vi "InstrumentCalibration - Remove Channel (SubVI).vi"(8 "error in":errorcluster, 11 "Table":string[][](array[string])) -> (0 "error out":errorcluster, 2 "Cancel out":bool, 3 "index":u16)   [LabVIEW 2019]
uses:
  Controls/FGV States.ctl
panel:
  in  "Cancel":bool
  in  "Ok":bool
  in  "Channel to Remove":u16(ring)
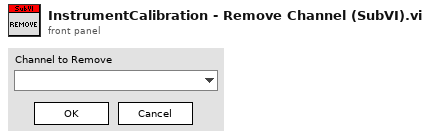
[diagram p1: front panel]
types:
  T1 = typedef "FGV States.ctl" = enum16{"Read", "Write"}
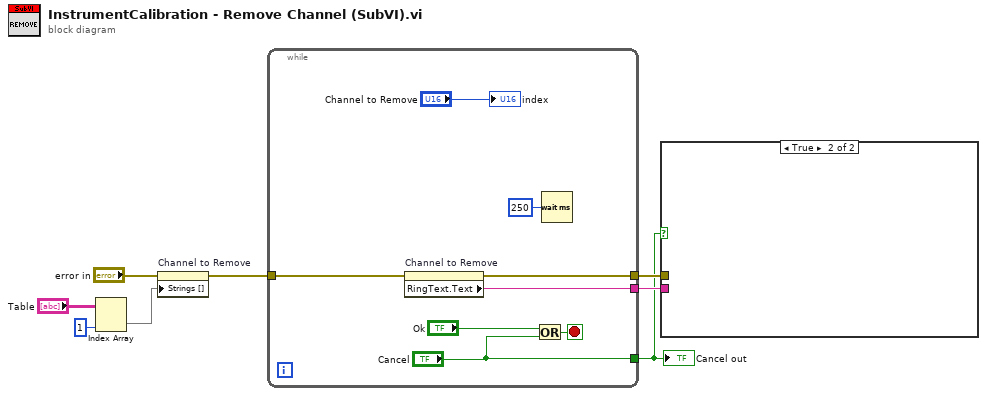
[diagram p0: block diagram]
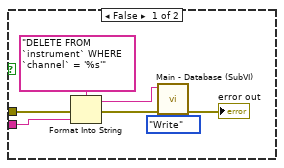
[diagram p2: hidden frame]
diagram:
  n1 = Index Array(array="Table", index (col)=1 ("disabled index (col)")) -> (element=w4:string[])  [unwired: 1 in]
  n2 = property on="Channel to Remove" class="Ring (strict)"(error in="error in", "Strings []"=w4) -> (error out=w7:errorcluster)  [unwired: 1 in, 1 out]
  n3 = while {
    tunnel: ["Cancel"] -> w1
    tunnel: [w11] -> w3
    tunnel: w7 -> [w10]
    tunnel: [w9] -> w2
    stop <- w14 stop-if-true
    n4 = property on="Channel to Remove" class="Ring (strict)"(error in=w10) -> (error out=w11:errorcluster, "RingText.Text"=w9:string)  [unwired: 1 in, 1 out]
    n5 = Or(x="Ok", y="Cancel") -> (x .or. y?=w14:bool)
    n6 = Wait (ms)(milliseconds to wait=u32 250) -> ()  [unwired: 1 out]
    "index" <- "Channel to Remove"
  }
  "Cancel out" <- w1
  n7 = case shown="True" w1 {
    tunnel: w3 -> [w21 _]
    tunnel: w2 -> [w19 _]
    frame False {
      n8 = Format Into String(format string="DELETE FROM `instrument` WHERE `channel` = '%s'" ("SQL query"), error in=w21, w19) -> (resulting string=w18:string, error out=w20:errorcluster)  [unwired: 1 in]
      n9 = call "Main - Database (SubVI).vi"("Enum"=FGV_States."Write", "error in (no error)"=w20, "SQL query"=w18) -> ("error out"=→"error out":errorcluster)  [unwired: 7 in, 1 out]
    }
    frame True {
    }
  }
